vi "Temperature Limit.vi"() -> ()   [LabVIEW 2015]
doc: "This VI simulates the acquisition of temperature, graphs the temperature, and notifies the user if the temperature is over the limit."
panel:
  in  "Start":bool
  in  "Delta t (ms)":i32(slide)=400 scale=50.0..500.0
  in  "Stop":bool
  in  "High Limit":dbl=28.0 format="%.2f"
  out "Temperature":cluster{"Temperature":dbl, "High Limit":dbl}(graph)={"Temperature"=85.88749999999999, "High Limit"=80.0}
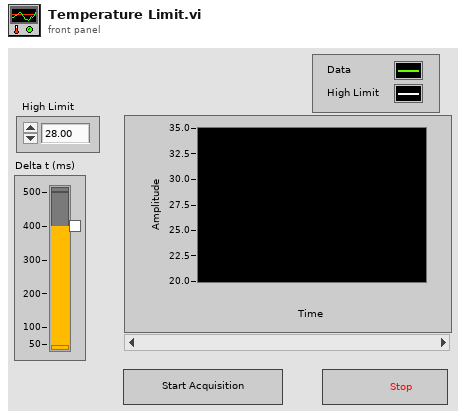
[diagram p1: front panel]
types:
  T1 = enum16{"Always On", "Always Off", "Off While Running"}
  T2 = cluster{"Temperature Value":dbl, "High Limit":dbl}
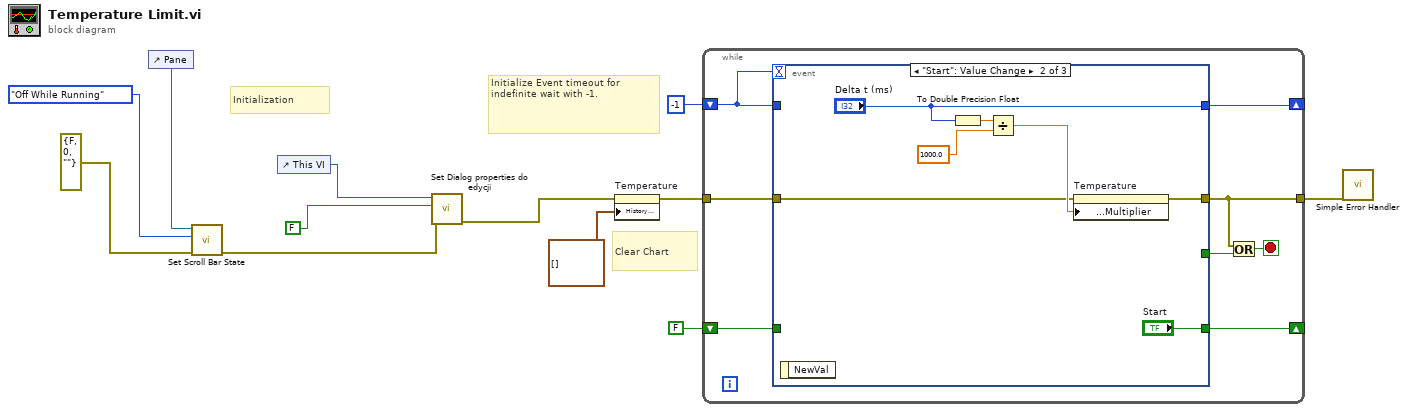
[diagram p0: block diagram]
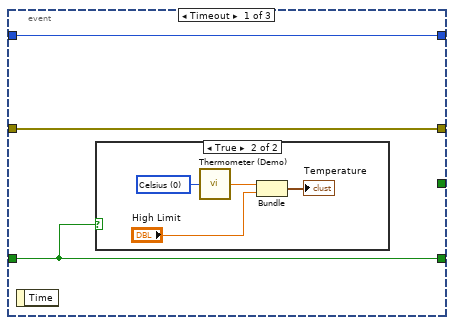
[diagram p2: hidden frame]
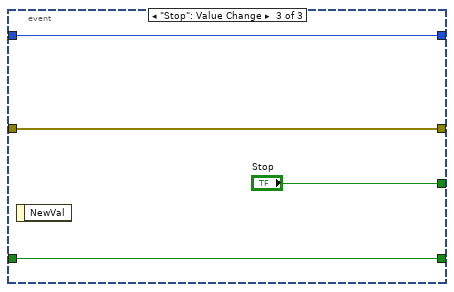
[diagram p4: hidden frame]
diagram:
  # "Clear Chart"
  # "Initialize Event timeout for indefinite wait with -1."
  # "Initialization"
  n1 = control-ref of="Pane"() -> (w2:refnum<vi>)
  n2 = call "Set Scroll Bar State.vi"("error in (no error)"=errorcluster {"status"=FALSE, "code"=0, "source"=""}, "Horizontal Scrollbar Visibility"=T1."Off While Running", "Pane Ref in"=w2) -> ("error out"=w5:errorcluster)  [unwired: 7 in, 1 out]
  n3 = control-ref of="This VI"() -> (w6:refnum<vi>)
  n4 = call "Set Dialog properties do edycji.vi"("error in (no error)"=w5, "Boolean"=FALSE, "VI in"=w6) -> ("error out"=w4:errorcluster)  [unwired: 8 in]
  n5 = property on="Temperature" class="WFChart (strict)"(error in=w4, "History Data"=cluster{"Temperature":dbl, "High Limit":dbl}[] []) -> (error out=w11:errorcluster)  [unwired: 1 in, 1 out]
  n6 = while {
    tunnel: w11 -> [w20]
    tunnel: [w18] -> w9
    shift-right: [w16] -> _
    shift-left: FALSE ("Start") -> [w15]
    shift-right: [w14] -> _
    shift-left: -1 ("Delta t (ms)") -> [w13]
    stop <- w19 stop-if-true
    n7 = event shown="[1] \"Start\": Value Change" {
      selector: _ -> [_ _ _]
      dyn-events: _ -> [_ _ _]
      timeout: w13 -> [_ _ _]
      tunnel: [_ _ "Stop"] -> w17
      tunnel: w20 -> [w23 w28 w37]
      tunnel: [w23 w34 w37] -> w18
      tunnel: [w21 "Start" w36] -> w16
      tunnel: w15 -> [w21 _ w36]
      tunnel: [w22 "Delta t (ms)" w35] -> w14
      tunnel: w13 -> [w22 _ w35]
      event Timeout {
        n8 = event-data() -> ()  [unwired: 1 in, 1 out]
        n9 = case shown="True" w21 {
          frame False {
          }
          frame True {
            w24 = u16 0 items=["Celsius", "Fahrenheit"] ("Units (0: Celsius)")
            n10 = call "Thermometer (Demo).vi"("Units (0: Celsius)"=w24) -> ("Temperature Value"=w25:dbl)
            n11 = Bundle("Temperature Value"=w25, "High Limit"="High Limit") -> (→"Temperature":T2)  [unwired: 1 in]
          }
        }
      }
      event "Start": Value Change {
        n12 = event-data() -> ()  [unwired: 1 in, 1 out]
        n13 = To Double Precision Float(number="Delta t (ms)") -> (double precision float=w33:dbl)
        n14 = Divide(x=w33, y=1000.0) -> (x/y=w31:dbl)
        n15 = property on="Temperature" class="WFChart (strict)"(error in=w28, "X Scale.Offset and Multiplier:Multiplier"=w31) -> (error out=w34:errorcluster)  [unwired: 1 in, 1 out]
      }
      event "Stop": Value Change {
        n16 = event-data() -> ()  [unwired: 1 in, 1 out]
      }
    }
    n17 = Or(x=w18, y=w17) -> (x .or. y?=w19:bool)
  }
  n18 = call <vilib>:"Simple Error Handler.vi"("error in (no error)"=w9) -> ()  [unwired: 4 in, 5 out]
